vi "test_Basic Host Api.vi"(8 "error in (no error)":errorcluster, 11 "TestCase in":refnum<class "Instrument Addon Host API Tests.lvclass">) -> (0 "error out":errorcluster, 3 "TestCase out":refnum<class "Instrument Addon Host API Tests.lvclass">)   [LabVIEW 2018, in "Instrument Addon Host API Tests.lvclass"]
uses:
  Instrument Addon Host API Tests.lvclass
  Addon/Addon Shared/Types/Buffered RT Instrument Command.ctl
  Addon/Addon Shared/Types/Response Wait Type.ctl
  <vilib>/addons/_JKI Toolkits/VI Tester/TestCase.llb/TestCase.lvclass
  APIs/Host Automation API/Instrument Host Automation API.lvlib
  Addon/Addon Shared/Instrument Addon Shared.lvlib
  C:/Program Files (x86)/National Instruments/LabVIEW 2018/vi.lib/addons/_JKI Toolkits/VI Tester/TestCase.llb/TestCase.lvclass
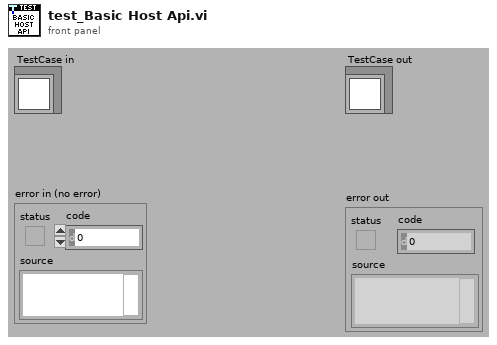
[diagram p1: front panel]
types:
  T1 = typedef "Instrument Addon Shared.lvlib/Buffered RT Instrument Command.ctl" = cluster{"Command":string, "Response Expected?":bool, "Wait Type":T2, "Wait Value":dbl}
  T2 = typedef "Instrument Addon Shared.lvlib/Response Wait Type.ctl" = enum16{"Byte Count", "Wait sec"}
  T3 = typedef "NI STM.lvlib/TCP Connection Info.ctl" = cluster{"connection ID":refnum<k5>, "meta data":T4[]}
  T4 = typedef "NI STM.lvlib/MetaDataElement.ctl" = string
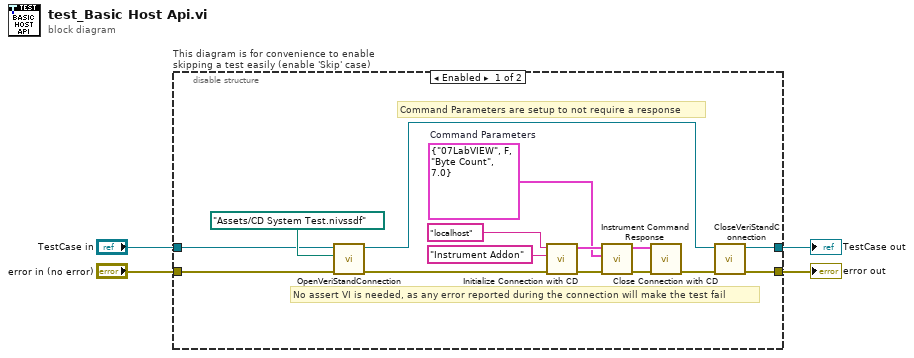
[diagram p0: block diagram]
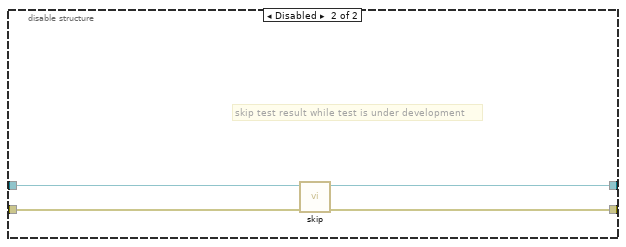
[diagram p2: hidden frame]
diagram:
  n1 = disable-structure "This diagram is for convenience to enable skipping a test easily (enable 'Skip' case)" shown="Enabled" {
    disable-tunnel: "TestCase in" -> [w10 w23]
    disable-tunnel: [w7 w21] -> w1
    disable-tunnel: [w8 w22] -> w3
    disable-tunnel: "error in (no error)" -> [w11 w20]
    frame Enabled {
      w15 = T1 {"Command"="07LabVIEW", "Response Expected?"=FALSE, "Wait Type"=enum."Byte Count", "Wait Value"=7.0}  # Command Parameters
      # "Command Parameters are setup to not require a response"
      # "No assert VI is needed, as any error reported during the connection will make the test fail"
      n2 = call-dynamic "OpenVeriStandConnection.vi"("error in (no error)"=w11, "System Definition File"=path "Assets/CD System Test.nivssdf", "VeriStand Test Case in"=w10) -> ("error out"=w5:errorcluster, "VeriStand Test Case out"=w6:refnum<class "Instrument Addon Host API Tests.lvclass">)  [unwired: 6 in, 1 out]
      n3 = call "Initialize Connection with CD.vi"("error in (no error)"=w5, "TCP Service"="Instrument Addon", "IP Address"="localhost") -> ("error out"=w17:errorcluster, "connection info out"=w16:T3)  [unwired: 7 in]
      n4 = call "Instrument Command Response.vi"("error in (no error)"=w17, "Command Parameters"=w15, "Comm.Info"=w16) -> ("error out"=w13:errorcluster, "Comm.Info"=w14:T3)  [unwired: 5 in, 2 out]
      n5 = call "Close Connection with CD.vi"("error in"=w13, "Comm.Info"=w14) -> ("error out"=w9:errorcluster)  [unwired: 9 in]
      n6 = call-dynamic "CloseVeriStandConnection.vi"("error in (no error)"=w9, "VeriStand Test Case in"=w6) -> ("error out"=w8:errorcluster, "VeriStand Test Case out"=w7:refnum<class "Instrument Addon Host API Tests.lvclass">)  [unwired: 8 in]
    }
    frame Disabled {
      # "skip test result while test is under development"
      n7 = call <vilib>:"skip.vi"("error in (no error)"=w20, "TestCase in"=w23) -> ("error out"=w22:errorcluster, "TestCase out"=w21:refnum<class "Instrument Addon Host API Tests.lvclass">)  [unwired: 8 in]
    }
  }
  "error out" <- w3
  "TestCase out" <- w1
